vi "Test_HW_Loop.vi"(7 "ErrorLocation":string="FPGA") -> (0 "error out":errorcluster, 2 "Probe 1":i16)   [LabVIEW 2018]
uses:
  Queue/DataQueueElements.ctl
  <vilib>/rvi/interface/nirviOpenFPGA/nirviOpenFPGA.xnode
  <vilib>/rvi/interface/nirviMethod/nirviMethod.xnode
  <vilib>/FPGAPlugInAG/Dynamic/niLvFpga_Reset_Dynamic.vi
  <vilib>/FPGAPlugInAG/Dynamic/niLvFpga_Run_Dynamic.vi
  <vilib>/FPGAPlugInAG/Dynamic/niLvFpga_ConfigureFifo_Dynamic.vi
  <vilib>/rvi/errors/niLvFpgaMergeErrorWithErrorCode.vi
  <vilib>/FPGAPlugInAG/Dynamic/niLvFpga_StartFifo_Dynamic.vi
  Controls/Clusts/FPGA_Scale.ctl
  Controls/Clusts/FreqShift.ctl
  Controls/Clusts/FP_UserTargetConfig.ctl
  Controls/Clusts/FrontPanel_UserConfig.ctl
  Controls/PathsCluster.ctl
  Controls/Clusts/UserConfig.ctl
  Controls/Clusts/Config_Clust.ctl
  Queue/HWQueueElements.ctl
  Controls/Enums/TargetNumber.ctl
  Controls/Clusts/AcqData.ctl
  <vilib>/FPGAPlugInAG/Dynamic/niLvFpga_ReadFifo_Dynamic.vi
  <vilib>/rvi/interface/nirviCloseFPGA/nirviCloseFPGA.xnode
  Controls/Clusts/FPGA_Config_Clust.ctl
  Controls/HWCluster.ctl
  Controls/Enums/NoiseQueueElements.ctl
  Controls/Enums/ScaleMeasure.ctl
  <vilib>/FPGAPlugInAG/Dynamic/niLvFpga_Close_Dynamic.vi
  <vilib>/rvi/interface/nirviReadWriteControl/nirviReadWriteControl.xnode
  Controls/RadioButtons/FilterEnableRadio.ctl
  Controls/Clusts/Inclinometer_User_Cfg.ctl
  ATA_Source_20180912/ATA_RF_Acq/FPGA Bitfiles/2018090501_10_ATA_Target1.lvbitx
  <vilib>/rvi/interface/Simulation/niFpgaSimulationCallBeginRW.vi
  <vilib>/rvi/errors/niLvFpgaAdjustHostInterfaceError.vi
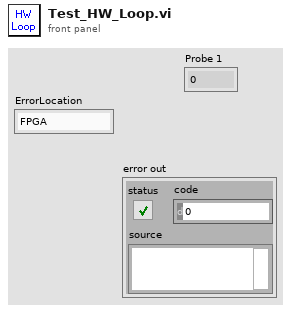
[diagram p1: front panel]
types:
  T1 = typedef "HWQueueElements.ctl" = enum16{"HW_Init", "HW_UpdtCfg", "HW_Start", "HW_Pause", "HW_Run", "HW_Cls", "HW_Exit"}
  T2 = typedef "HWCluster.ctl" = cluster{"FPGA":T3}
  T3 = typedef "FPGA_Config_Clust.ctl" = cluster{"Target":T4, "Channel":T4, "Ref1":refnum<k20>, "Ref2":refnum<k20>}
  T4 = typedef "TargetNumber.ctl" = enum16{"1", "2", "3", "4"}
  T5 = typedef "NoiseQueueElements.ctl" = enum16{"Noise_Startup", "Noise_Init", "Noise_Macro", "Noise_Config", "Noise_NewData", "Noise_Transform", "Noise_SumdTrace", "Noise_Send", "Noise_Probes", "Noise_Exit"}
  T6 = typedef "DataQueueElements.ctl" = enum16{"Data_Init", "Data_Config", "Data_AddData", "Data_FreqShift", "Data_FPGA_Write", "Data_Transform", "Data_Send", "Data_Exit"}
  T7 = enum8{"Internal Clock PLL Off", "Internal Clock PLL On (CLK_IN)", "External Clock (CLK_IN)", "Internal Clock PLL On (IoModSyncClk)"}
  T8 = typedef "Config_Clust.ctl" = cluster{"UsrCfg":T9, "FP_User":T11}
  T9 = typedef "UserConfig.ctl" = cluster{"Paths":T10, "SampleRate":dbl}
  T10 = typedef "PathsCluster.ctl" = cluster{"CfgFile":path, "LogFolder":path, "LogFile":path, "NAS path":path, "ThreshFile":path, "RedunFolder":path}
  T11 = typedef "FrontPanel_UserConfig.ctl" = cluster{"#NoiseSums":u32, "Max_df":u32, "AvgAvg":bool, "#Avg":u16, "AutoCenter":bool, "Inclin":T12, "1":T13, "2":T13, "3":T13, "4":T13, "Target to Probe":T4, "SNR_Thresh":dbl, "Paths":T10, "Connex_Location":string, "SimulateFPGA":bool}
  T12 = typedef "Inclinometer_User_Cfg.ctl" = cluster{"Vmin":dbl, "Vmax":dbl, "Angle_min":dbl, "Angle_max":dbl, "Offset":dbl, "Pos_Neg":bool}
  T13 = typedef "FP_UserTargetConfig.ctl" = cluster{"Cal_":T14, "Beac":T14, "Scale":T15, "Offset":fxp<+/-,16,16>, "Scale_Noise":fxp<+/-,30,30>, "Scale_Step1":fxp<+/-,17,17>, "Scale_In_RT":ext, "ScaleMeas":fxp<+/-,16,1>, "FreqsToRemove":i32[], "Width":i32[], "ScaleMeasEnum":T16, "FilterEnab":T17}
  T14 = typedef "FreqShift.ctl" = cluster{"Fine":dbl, "Coarse_":dbl}
  T15 = typedef "FPGA_Scale.ctl" = cluster{"Step4":fxp<+/-,23,23>, "Step5":fxp<+/-,23,23>, "Step6":fxp<+/-,23,23>, "Step7":fxp<+/-,23,23>}
  T16 = typedef "ScaleMeasure.ctl" = enum16{"1", "10", "50", "42"}
  T17 = typedef "FilterEnableRadio.ctl" = enum32{"None", "Step 1", "Frequency Shift", "Step 4", "Step 5", "Step 6", "Step 7"}
  T18 = typedef "AcqData.ctl" = cluster{"Data":fxp<+/-,24,1>[], "#":T4, "MeasMean":dbl, "1_Max":dbl, "4_Max":dbl, "5_Max":dbl, "6_Max":dbl, "7_Max":dbl}
  T19 = typedef "Semaphore RefNum" = refnum<k1>
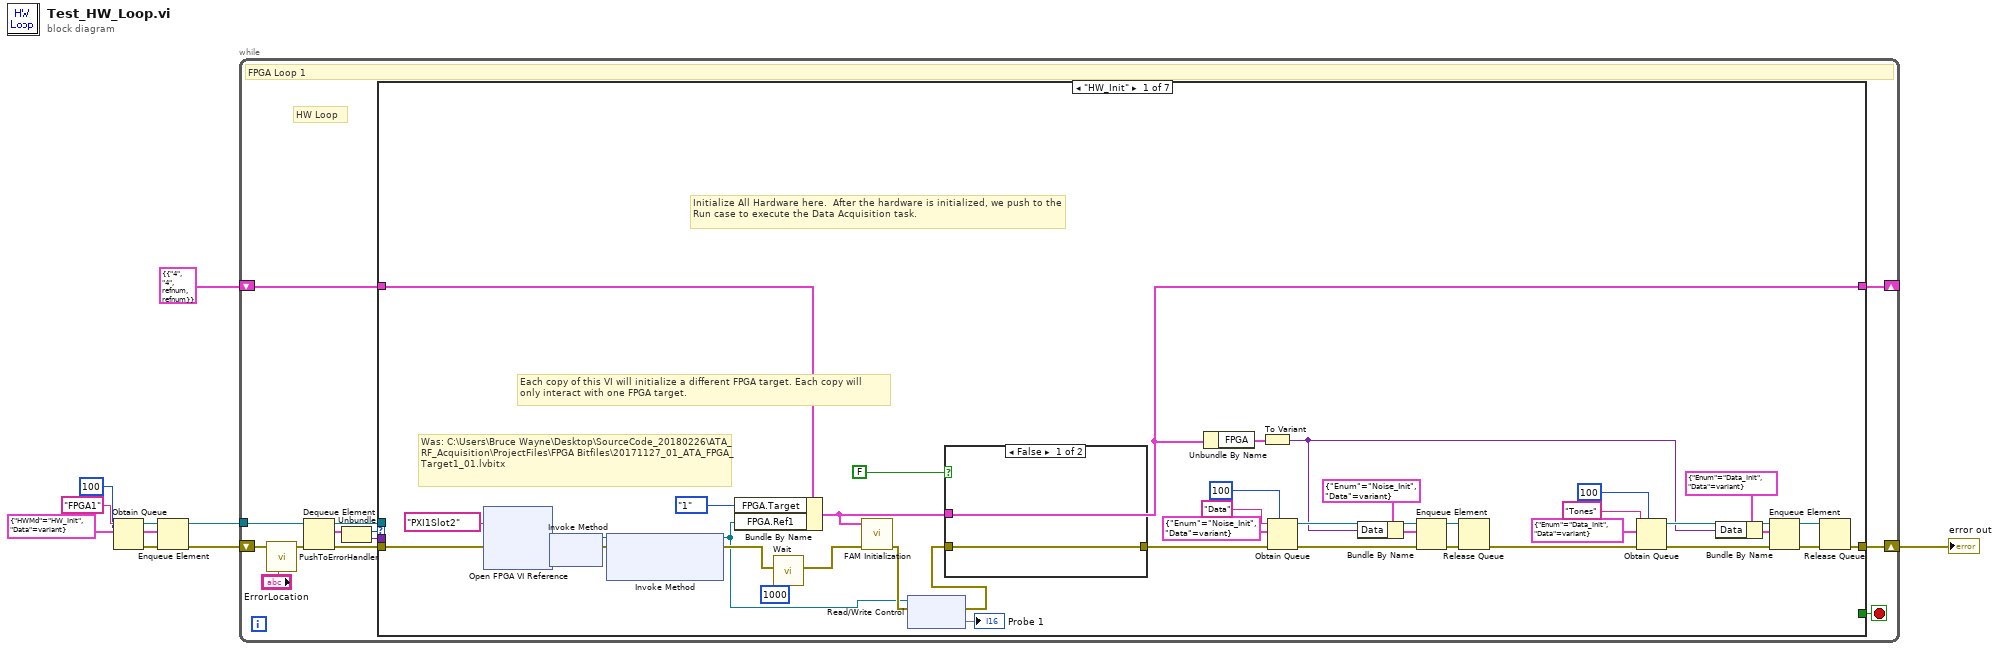
[diagram p0: block diagram]
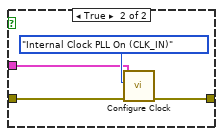
[diagram p2: hidden frame]
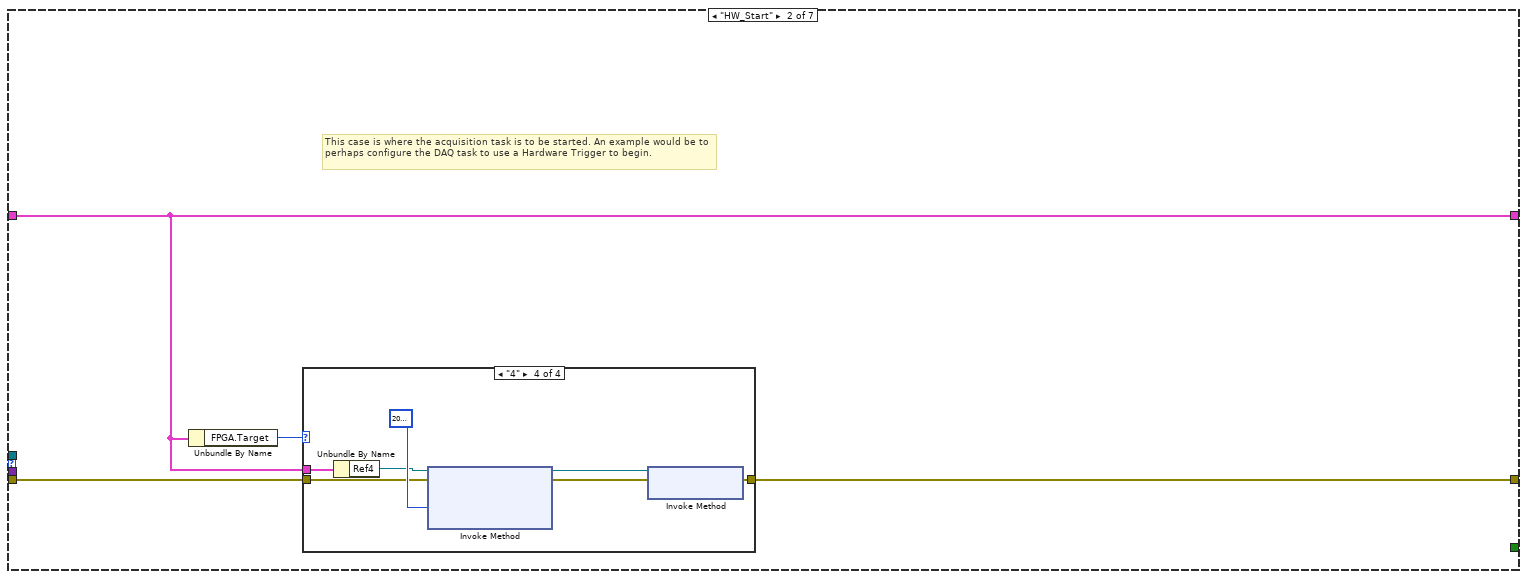
[diagram p3: hidden frame]
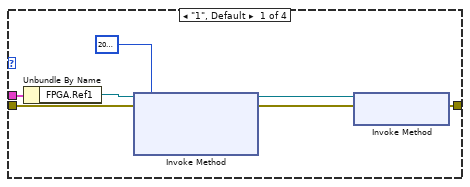
[diagram p4: hidden frame]
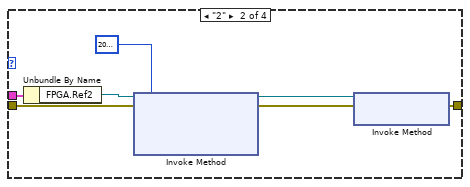
[diagram p5: hidden frame]
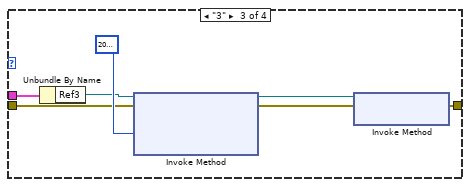
[diagram p6: hidden frame]
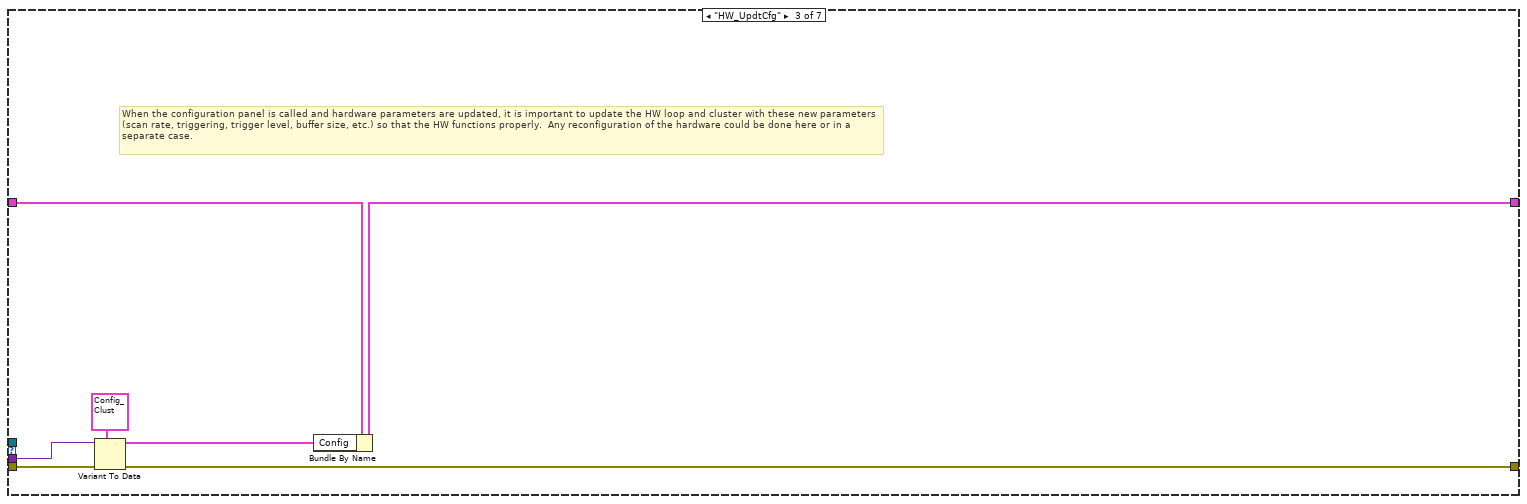
[diagram p7: hidden frame]
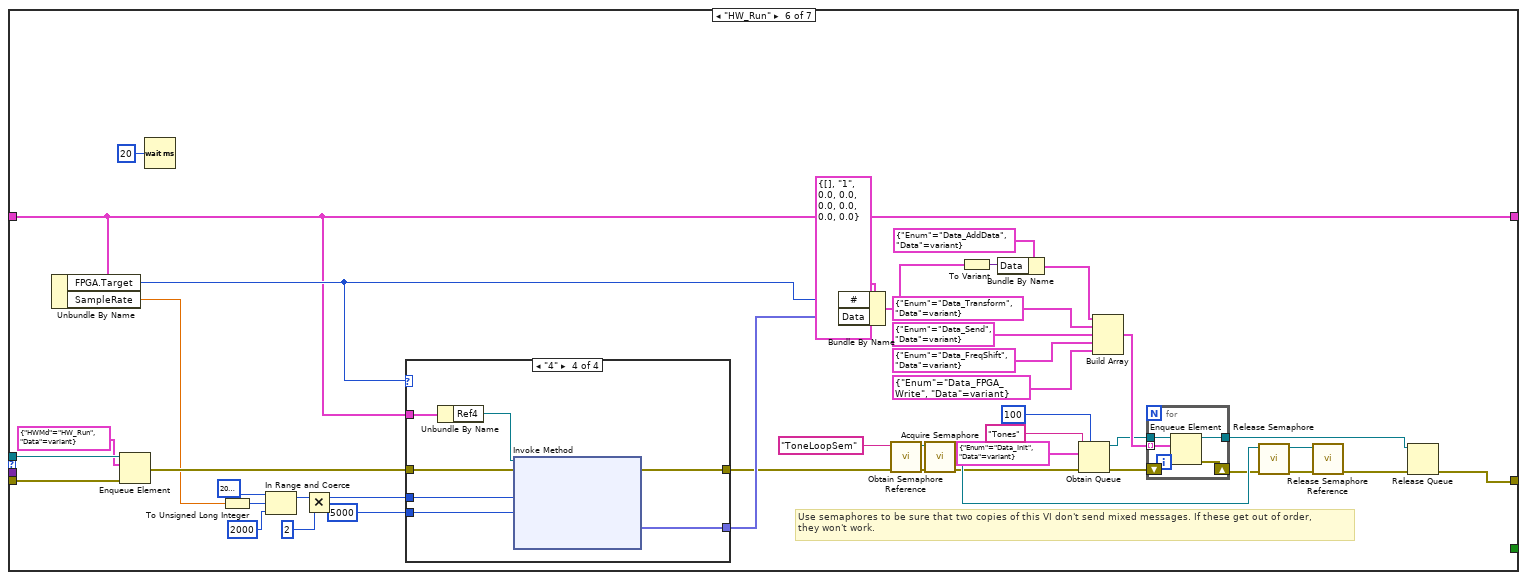
[diagram p10: hidden frame]
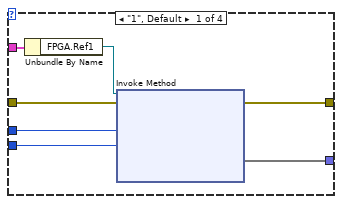
[diagram p11: hidden frame]
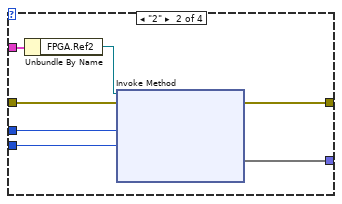
[diagram p12: hidden frame]
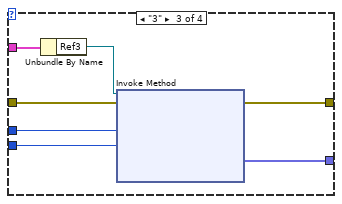
[diagram p13: hidden frame]
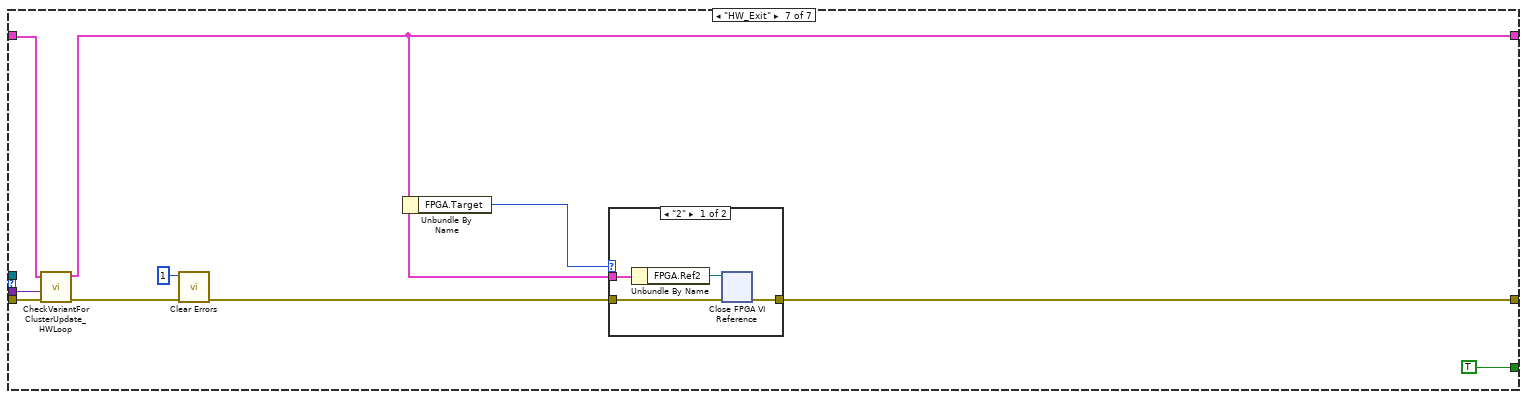
[diagram p14: hidden frame]
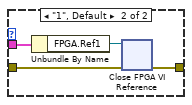
[diagram p15: hidden frame]
diagram:
  w1 = cluster{"HWMd":T1, "Data":variant} {"HWMd"=enum."HW_Init", "Data"=variant}
  n1 = Obtain Queue(max queue size (-1, unlimited)=100, name (unnamed)="FPGA1", element data type=w1) -> (queue out=w5:refnum<queue>, error out=w3:errorcluster)  [unwired: 2 in, 1 out]
  n2 = Enqueue Element(queue=w5, element=w1, error in (no error)=w3) -> (queue out=w4:refnum<queue>, error out=w2:errorcluster)  [unwired: 1 in, 1 out]
  n3 = while {
    shift-right: [w11] -> w8
    shift-left: w2 -> [w13]
    shift-right: [w22] -> _
    shift-left: T2 {"FPGA"={"Target"=enum."4", "Channel"=enum."4", "Ref1"=refnum, "Ref2"=refnum}} ("ClusterOut") -> [w18]
    tunnel: w4 -> [w21]
    stop <- w14 stop-if-true
    # "HW Loop"
    # "FPGA Loop 1"
    n4 = call "PushToErrorHandler.vi"("ErrorIn"=w13, "ErrorLocation"="ErrorLocation") -> ("ErrorOut"=w12:errorcluster)  [unwired: 5 in]
    n5 = Dequeue Element(queue=w21, error in (no error)=w12) -> (queue out=w16:refnum<queue>, element=w20:cluster{"HWMd":T1, "Data":variant}, error out=w17:errorcluster)  [unwired: 2 out]
    n6 = Unbundle(w20) -> ("HWMd"=w19:T1, "Data"=w15:variant)
    n7 = case shown="\"HW_Init\"" w19 {
      tunnel: [w37 w70 w103 w108 w110 w112 w191] -> w11
      tunnel: [w42 w69 w105 w107 w109 w117 w188] -> w22
      tunnel: w18 -> [w44 w69 w106 w107 w109 w117 w194]
      tunnel: w17 -> [w62 w71 w104 w108 w110 w153 w195]
      tunnel: w16 -> [_ _ _ _ _ w152 _]
      tunnel: w15 -> [_ _ w102 _ _ _ w196]
      tunnel: [_ _ _ _ _ _ TRUE ("Exit?")] -> w14
      frame "HW_Init" {
        # "Was: C:\\Users\\Bruce Wayne\\Desktop\\SourceCode_20180226\\ATA_RF_Acquisition\\ProjectFiles\\FPGA Bitfiles\\20171127_01_ATA_FPGA_Target1_01.lvbitx"
        # "Each copy of this VI will initialize a different FPGA target. Each copy will\nonly interact with one FPGA target."
        # "Initialize All Hardware here.  After the hardware is initialized, we push to the Run case to execute the Data Acquisition task."
        n8 = xnode ("Open FPGA VI Reference")("error in"=w62, "resource name"=tag "PXI1Slot2") -> ("FPGA VI Reference Out"=w34:refnum<k20>, "error out"=w32:errorcluster)
        n9 = xnode "Invoke Method"("FPGA VI Reference In"=w34, "error in"=w32) -> ("FPGA VI Reference Out"=w33:refnum<k20>, "error out"=w31:errorcluster)
        n10 = xnode "Invoke Method"("FPGA VI Reference In"=w33, "error in"=w31) -> ("FPGA VI Reference Out"=w23:refnum<k20>, "error out"=w28:errorcluster)  [unwired: 1 in]
        n11 = Bundle By Name(cluster=w44, "FPGA.Target"=TargetNumber."1", "FPGA.Ref1"=w23) -> (w42:T2)
        n12 = call "Wait.vi"("Wait (ms)"=u32 1000, "ErrorIn"=w28) -> ("ErrorOut"=w27:errorcluster)  [unwired: 9 in]
        n13 = call "FAM Initialization.vi"("error in (no error)"=w27, "Cluster"=w42) -> ("error out"=w25:errorcluster)  [unwired: 8 in, 1 out]
        n14 = xnode "Read/Write Control"("FPGA VI Reference In"=w23, "error in"=w25) -> ("error out"=w24:errorcluster, "Probe 1"=→"Probe 1")  [unwired: 1 out]
        n15 = case shown="False" FALSE ("10MHzPLL?") {
          tunnel: w24 -> [w63 w66]
          tunnel: [w63 w65] -> w43
          tunnel: w42 -> [_ w64]
          frame False {
          }
          frame True {
            n16 = call "Configure Clock.vi"("error in"=w66, "Clock Source"=T7."Internal Clock PLL On (CLK_IN)", "Cluster"=w64) -> ("error out"=w65:errorcluster)  [unwired: 7 in, 1 out]
          }
        }
        n17 = Unbundle By Name(w42) -> ("FPGA"=w50:T3)
        n18 = To Variant(anything=w50) -> (Variant=w46:variant)
        n19 = Obtain Queue(max queue size (-1, unlimited)=100, name (unnamed)="Data", element data type=cluster{"Enum":T5, "Data":variant} {"Enum"=enum."Noise_Init", "Data"=variant}, error in (no error)=w43) -> (queue out=w49:refnum<queue>, error out=w51:errorcluster)  [unwired: 1 in, 1 out]
        n20 = Bundle By Name(cluster=cluster{"Enum":T5, "Data":variant} {"Enum"=enum."Noise_Init", "Data"=variant} ("element"), "Data"=w46) -> (w47:cluster{"Enum":T5, "Data":variant})
        n21 = Enqueue Element(queue=w49, element=w47, error in (no error)=w51) -> (queue out=w39:refnum<queue>, error out=w41:errorcluster)  [unwired: 2 out]
        n22 = Release Queue(queue=w39, error in (no error)=w41) -> (error out=w40:errorcluster)  [unwired: 1 in, 2 out]
        n23 = Obtain Queue(max queue size (-1, unlimited)=100, name (unnamed)="Tones", element data type=cluster{"Enum":T6, "Data":variant} {"Enum"=enum."Data_Init", "Data"=variant}, error in (no error)=w40) -> (queue out=w55:refnum<queue>, error out=w56:errorcluster)  [unwired: 1 in, 1 out]
        n24 = Bundle By Name(cluster=cluster{"Enum":T6, "Data":variant} {"Enum"=enum."Data_Init", "Data"=variant} ("element"), "Data"=w46) -> (w60:cluster{"Enum":T6, "Data":variant})
        n25 = Enqueue Element(queue=w55, element=w60, error in (no error)=w56) -> (queue out=w36:refnum<queue>, error out=w38:errorcluster)  [unwired: 2 out]
        n26 = Release Queue(queue=w36, error in (no error)=w38) -> (error out=w37:errorcluster)  [unwired: 1 in, 2 out]
      }
      frame "HW_Start" {
        # "This case is where the acquisition task is to be started. An example would be to perhaps configure the DAQ task to use a Hardware Trigger to begin."
        n27 = Unbundle By Name(w69) -> ("FPGA.Target"=w68:T4)
        n28 = case shown="\"4\"" w68 {
          tunnel: w69 -> [w75 w82 w89 w96]
          tunnel: w71 -> [w73 w80 w87 w94]
          tunnel: [w72 w79 w86 w93] -> w70
          frame "1", Default {
            n29 = Unbundle By Name(w75) -> ("FPGA.Ref1"=w74:refnum<k20>)
            n30 = xnode "Invoke Method"("FPGA VI Reference In"=w74, "error in"=w73, "Requested Depth"=u32 2000000 ("Num Samples")) -> ("FPGA VI Reference Out"=w76:refnum<k20>, "error out"=w77:errorcluster)  [unwired: 1 out]
            n31 = xnode "Invoke Method"("FPGA VI Reference In"=w76, "error in"=w77) -> ("error out"=w72:errorcluster)  [unwired: 1 out]
          }
          frame "2" {
            n32 = Unbundle By Name(w82) -> ("FPGA.Ref2"=w81:refnum<k20>)
            n33 = xnode "Invoke Method"("FPGA VI Reference In"=w81, "error in"=w80, "Requested Depth"=u32 2000000 ("Num Samples")) -> ("FPGA VI Reference Out"=w83:refnum<k20>, "error out"=w84:errorcluster)  [unwired: 1 out]
            n34 = xnode "Invoke Method"("FPGA VI Reference In"=w83, "error in"=w84) -> ("error out"=w79:errorcluster)  [unwired: 1 out]
          }
          frame "3" {
            n35 = Unbundle By Name(w89) -> ("Ref3"=w88:refnum<k20>)
            n36 = xnode "Invoke Method"("FPGA VI Reference In"=w88, "error in"=w87, "Requested Depth"=u32 2000000 ("Num Samples")) -> ("FPGA VI Reference Out"=w90:refnum<k20>, "error out"=w91:errorcluster)  [unwired: 1 out]
            n37 = xnode "Invoke Method"("FPGA VI Reference In"=w90, "error in"=w91) -> ("error out"=w86:errorcluster)  [unwired: 1 out]
          }
          frame "4" {
            n38 = Unbundle By Name(w96) -> ("Ref4"=w95:refnum<k20>)
            n39 = xnode "Invoke Method"("FPGA VI Reference In"=w95, "error in"=w94, "Requested Depth"=u32 2000000 ("Num Samples")) -> ("FPGA VI Reference Out"=w97:refnum<k20>, "error out"=w98:errorcluster)  [unwired: 1 out]
            n40 = xnode "Invoke Method"("FPGA VI Reference In"=w97, "error in"=w98) -> ("error out"=w93:errorcluster)  [unwired: 1 out]
          }
        }
      }
      frame "HW_UpdtCfg" {
        # "When the configuration panel is called and hardware parameters are updated, it is important to update the HW loop and cluster with these new parameters (scan rate, triggering, trigger level, buffer size, etc.) so that the HW functions properly.  Any reconfiguration of the hardware could be done here or in a separate case."
        n41 = Variant To Data(error in=w104, type=T8 {"UsrCfg"={"Paths"={"CfgFile"=path "", "LogFolder"=path "", "LogFile"=path "", "NAS path"=path "", "ThreshFile"=path "", "RedunFolder"=path ""}, "SampleRate"=12500.0}, "FP_User"={"#NoiseSums"=1, "Max_df"=1, "AvgAvg"=FALSE, "#Avg"=1, "AutoCenter"=FALSE, "Inclin"={"Vmin"=0.0, "Vmax"=0.0, "Angle_min"=0.0, "Angle_max"=0.0, "Offset"=0.0, "Pos_Neg"=FALSE}, "1"={"Cal_"={"Fine"=0.000213623046875, "Coarse_"=4194303.0}, "Beac"={"Fine"=4194303.0, "Coarse_"=1.0}, "Scale"={"Step4"=10000.0, "Step5"=4194303.0, "Step6"=1.0, "Step7"=10000.0}, "Offset"=0.0, "Scale_Noise"=4194303.0, "Scale_Step1"=65535.0, "Scale_In_RT"=1.0, "ScaleMeas"=0.999969482421875, "FreqsToRemove"=[0, 1633], "Width"=[0, 1633], "ScaleMeasEnum"=enum."50", "FilterEnab"=enum."Step 1"}, "2"={"Cal_"={"Fine"=0.000213623046875, "Coarse_"=4194303.0}, "Beac"={"Fine"=0.000213623046875, "Coarse_"=4194303.0}, "Scale"={"Step4"=0.0, "Step5"=4194303.0, "Step6"=1.0, "Step7"=10000.0}, "Offset"=0.0, "Scale_Noise"=4194303.0, "Scale_Step1"=65535.0, "Scale_In_RT"=1.0, "ScaleMeas"=0.999969482421875, "FreqsToRemove"=[0, 1633], "Width"=[0, 1633], "ScaleMeasEnum"=enum."50", "FilterEnab"=enum."Step 1"}, "3"={"Cal_"={"Fine"=0.000213623046875, "Coarse_"=4194303.0}, "Beac"={"Fine"=0.000213623046875, "Coarse_"=4194303.0}, "Scale"={"Step4"=0.0, "Step5"=4194303.0, "Step6"=1.0, "Step7"=10000.0}, "Offset"=0.0, "Scale_Noise"=4194303.0, "Scale_Step1"=65535.0, "Scale_In_RT"=1.0, "ScaleMeas"=0.999969482421875, "FreqsToRemove"=[0, 1633], "Width"=[0, 1633], "ScaleMeasEnum"=enum."50", "FilterEnab"=enum."Step 1"}, "4"={"Cal_"={"Fine"=0.000213623046875, "Coarse_"=4194303.0}, "Beac"={"Fine"=0.000213623046875, "Coarse_"=4194303.0}, "Scale"={"Step4"=0.0, "Step5"=4194303.0, "Step6"=1.0, "Step7"=10000.0}, "Offset"=0.0, "Scale_Noise"=4194303.0, "Scale_Step1"=1.0, "Scale_In_RT"=10000.0, "ScaleMeas"=0.999969482421875, "FreqsToRemove"=[0, 1633], "Width"=[0, 1633], "ScaleMeasEnum"=enum."50", "FilterEnab"=enum."Step 1"}, "Target to Probe"=enum."4", "SNR_Thresh"=1.0, "Paths"={"CfgFile"=path "", "LogFolder"=path "", "LogFile"=path "", "NAS path"=path "", "ThreshFile"=path "", "RedunFolder"=path ""}, "Connex_Location"="", "SimulateFPGA"=FALSE}} ("Config"), Variant=w102) -> (data=w101:T8, error out=w103:errorcluster)
        n42 = Bundle By Name(cluster=w106, "Config"=w101) -> (w105:T2)
      }
      frame "HW_Cls" {
        # "Close All Hardware"
      }
      frame "HW_Pause" {
      }
      frame "HW_Run" {
        # "Use semaphores to be sure that two copies of this VI don't send mixed messages. If these get out of order,\nthey won't work."
        n43 = Unbundle By Name(w117) -> ("FPGA.Target"=w118:T4, "SampleRate"=w142:dbl)
        n44 = Enqueue Element(queue=w152, element=cluster{"HWMd":T1, "Data":variant} {"HWMd"=enum."HW_Run", "Data"=variant}, error in (no error)=w153) -> (error out=w143:errorcluster)  [unwired: 3 out]
        n45 = Wait (ms)(milliseconds to wait=u32 20) -> ()  [unwired: 1 out]
        n46 = To Unsigned Long Integer(number=w142) -> (unsigned 32bit integer=w149:u32)
        n47 = In Range and Coerce(upper limit=u32 2000000 ("Num Samples"), x=w149, lower limit=u32 2000) -> (coerced(x)=w147:u32)  [unwired: 1 out]
        n48 = Multiply(x=w147, y=u32 2) -> (x*y=w150:u32)
        n49 = case shown="\"4\"" w118 {
          tunnel: w150 -> [w160 w167 w174 w181]
          tunnel: 5000 ("Timeout (ms)") -> [w159 w166 w173 w180]
          tunnel: w143 -> [w158 w165 w172 w179]
          tunnel: [w157 w164 w171 w178] -> w136
          tunnel: [w156 w163 w170 w177] -> w116
          tunnel: w117 -> [w154 w161 w168 w175]
          frame "1", Default {
            n50 = Unbundle By Name(w154) -> ("FPGA.Ref1"=w155:refnum<k20>)
            n51 = xnode "Invoke Method"("FPGA VI Reference In"=w155, "error in"=w158, "Number of Elements"=w160, "Timeout (ms)"=w159) -> ("error out"=w156:errorcluster, "Data"=w157:void[])  [unwired: 2 out]
          }
          frame "2" {
            n52 = Unbundle By Name(w161) -> ("FPGA.Ref2"=w162:refnum<k20>)
            n53 = xnode "Invoke Method"("FPGA VI Reference In"=w162, "error in"=w165, "Number of Elements"=w167, "Timeout (ms)"=w166) -> ("error out"=w163:errorcluster, "Data"=w164:void[])  [unwired: 2 out]
          }
          frame "3" {
            n54 = Unbundle By Name(w168) -> ("Ref3"=w169:refnum<k20>)
            n55 = xnode "Invoke Method"("FPGA VI Reference In"=w169, "error in"=w172, "Number of Elements"=w174, "Timeout (ms)"=w173) -> ("error out"=w170:errorcluster, "Data"=w171:fxp<+/-,40,1>[])  [unwired: 2 out]
          }
          frame "4" {
            n56 = Unbundle By Name(w175) -> ("Ref4"=w176:refnum<k20>)
            n57 = xnode "Invoke Method"("FPGA VI Reference In"=w176, "error in"=w179, "Number of Elements"=w181, "Timeout (ms)"=w180) -> ("error out"=w177:errorcluster, "Data"=w178:fxp<+/-,40,1>[])  [unwired: 2 out]
          }
        }
        n58 = Bundle By Name(cluster=T18 {"Data"=[], "#"=enum."1", "MeasMean"=0.0, "1_Max"=0.0, "4_Max"=0.0, "5_Max"=0.0, "6_Max"=0.0, "7_Max"=0.0}, "#"=w118, "Data"=w136) -> (w135:T18)
        n59 = call <vilib>:"Obtain Semaphore Reference.vi"("error in (no error)"=w116, "name (unnamed)"="ToneLoopSem") -> ("error out"=w125:errorcluster, "semaphore"=w127:T19)  [unwired: 3 in, 1 out]
        n60 = call <vilib>:"Acquire Semaphore.vi"("error in (no error)"=w125, "semaphore"=w127) -> ("error out"=w115:errorcluster, "semaphore out"=w126:T19)  [unwired: 3 in, 1 out]
        n61 = To Variant(anything=w135) -> (Variant=w139:variant)
        n62 = Bundle By Name(cluster=cluster{"Enum":T6, "Data":variant} {"Enum"=enum."Data_AddData", "Data"=variant}, "Data"=w139) -> (w140:cluster{"Enum":T6, "Data":variant})
        n63 = Obtain Queue(max queue size (-1, unlimited)=100, name (unnamed)="Tones", element data type=cluster{"Enum":T6, "Data":variant} {"Enum"=enum."Data_Init", "Data"=variant}, error in (no error)=w115) -> (queue out=w121:refnum<queue>, error out=w114:errorcluster)  [unwired: 1 in, 1 out]
        n64 = Build Array(w140, cluster{"Enum":T6, "Data":variant} {"Enum"=enum."Data_Transform", "Data"=variant}, cluster{"Enum":T6, "Data":variant} {"Enum"=enum."Data_Send", "Data"=variant}, cluster{"Enum":T6, "Data":variant} {"Enum"=enum."Data_FreqShift", "Data"=variant}, cluster{"Enum":T6, "Data":variant} {"Enum"=enum."Data_FPGA_Write", "Data"=variant}) -> (w122:cluster{"Enum":T6, "Data":variant}[])
        n65 = for {
          tunnel: w121 -> [w184]
          tunnel: w122 -> [w183] mode=indexing
          shift-right: [w185] -> w123
          shift-left: w114 -> [w186]
          tunnel: [w182] -> w111
          n66 = Enqueue Element(queue=w184, element=w183, error in (no error)=w186) -> (queue out=w182:refnum<queue>, error out=w185:errorcluster)  [unwired: 1 in, 1 out]
        }
        n67 = call <vilib>:"Release Semaphore.vi"("error in (no error)"=w123, "semaphore"=w126) -> ("error out"=w124:errorcluster, "semaphore out"=w120:T19)  [unwired: 4 in]
        n68 = call <vilib>:"Release Semaphore Reference.vi"("error in (no error)"=w124, "semaphore"=w120) -> ("error out"=w113:errorcluster)  [unwired: 8 in, 1 out]
        n69 = Release Queue(queue=w111, error in (no error)=w113) -> (error out=w112:errorcluster)  [unwired: 1 in, 2 out]
      }
      frame "HW_Exit" {
        n70 = call "CheckVariantForClusterUpdate_HWLoop.vi"("ErrorIn"=w195, "VariantIn"=w196, "ClusterIn"=w194) -> ("ErrorOut"=w192:errorcluster, "ClusterOut"=w188:T2)  [unwired: 7 in]
        n71 = call <vilib>:"Clear Errors.vi"("error in (no error)"=w192, "specific error code to clear (0: all)"=1) -> ("error out"=w190:errorcluster)  [unwired: 4 in, 1 out]
        n72 = Unbundle By Name(w188) -> ("FPGA.Target"=w187:T4)
        n73 = case shown="\"2\"" w187 {
          tunnel: [w200 w204] -> w191
          tunnel: w190 -> [w198 w202]
          tunnel: w188 -> [w197 w201]
          frame "2" {
            n74 = Unbundle By Name(w197) -> ("FPGA.Ref2"=w199:refnum<k20>)
            n75 = xnode ("Close FPGA VI Reference")("FPGA VI Reference In"=w199, "error in"=w198) -> ("error out"=w200:errorcluster)
          }
          frame "1", Default {
            n76 = Unbundle By Name(w201) -> ("FPGA.Ref1"=w203:refnum<k20>)
            n77 = xnode ("Close FPGA VI Reference")("FPGA VI Reference In"=w203, "error in"=w202) -> ("error out"=w204:errorcluster)
          }
        }
      }
    }
  }
  "error out" <- w8
